vi "RSNRPZ Get Scope Measurements Pulse Transition.vi"(8 "error in (no error)":errorcluster, 9 "Slope (0: Positive)":i32(ring) items=["Positive", "Negative"], 10 "Channel (1)":i32=1, 11 "VISA session":refnum<visa-resource-name> caption="VISA resource name") -> (0 "error out":errorcluster, 1 "Duration":dbl format="%^.3e", 3 "dup VISA session":refnum<visa-resource-name> caption="VISA resource name", 4 "Occurence":dbl format="%^.3e", 5 "Overshoot":dbl format="%^.3e")   [LabVIEW 2010]
doc: "This VI returns the transition parameters of the last examined trace data.\nThe NRP Sensor always searches for the first rising edge and the first falling edge in the trace. If offset time is set greater than zero the algorithm searches the edges from this time in the trace.\n\nNote:\n1) This VI is only available for NRP-Z81.\n\nRemote-control command(s):\nSENS:TRAC:MEAS:TRAN:POS:DUR?\nSENS:TRAC:MEAS:TRAN:POS:OCC?\nSENS:TRAC:MEAS:TRAN:POS:OVER?\nSENS:TRAC:MEAS:TRAN:NEG:DUR?\nSENS:TRAC:MEAS:TRAN:NEG:OCC?\nSENS:TRAC:MEAS:TRAN:NEG:OVER?"
uses:
  rsnrpz_32.dll
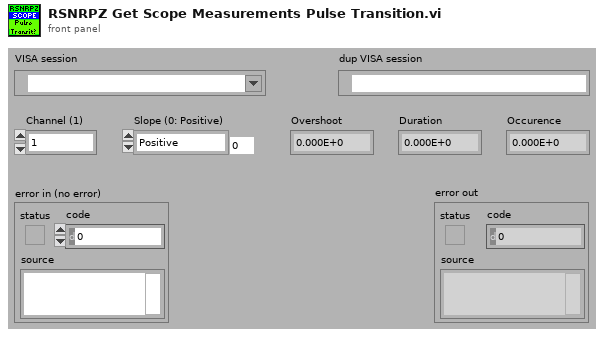
[diagram p1: front panel]
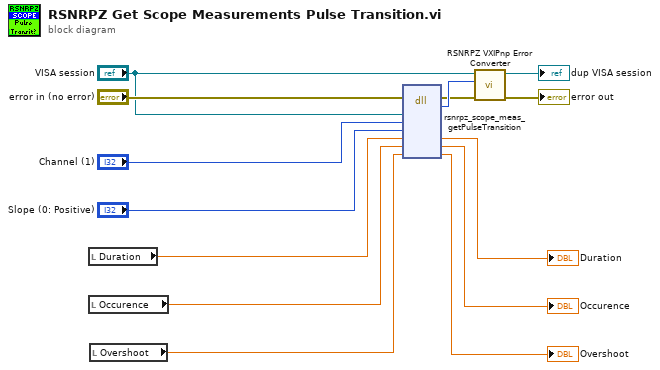
[diagram p0: block diagram]
diagram:
  n1 = local read "Duration"() -> (w11:dbl)
  n2 = local read "Occurence"() -> (w9:dbl)
  n3 = local read "Overshoot"() -> (w7:dbl)
  n4 = dll-call lib="rsnrpz_32.dll" fn="rsnrpz_scope_meas_getPulseTransition"(error in="error in (no error)", "Instrument Handle"="VISA session", "Channel"="Channel (1)", "Slope"="Slope (0: Positive)", "Duration"=w11, "Occurence"=w9, "Overshoot"=w7) -> (error out=w5:errorcluster, "Status"=w14:i32, "Duration"=→"Duration":dbl, "Occurence"=→"Occurence":dbl, "Overshoot"=→"Overshoot":dbl)  [unwired: 5 in, 1 out]
  n5 = call <instrlib>:"RSNRPZ VXIPnp Error Converter.vi"("error in"=w5, "VXIPnp error code"=w14, "VISA session"="VISA session") -> ("error out"=→"error out":errorcluster, "dup VISA session"=→"dup VISA session":refnum<visa-resource-name>)  [unwired: 7 in]
